vi "Check Large Range.vi"(8 "Tolerance":dbl=20.0, 9 "Differential Pressure":dbl, 10 "Diff Press Setpoint":dbl) -> (1 "In Range?":bool)   [LabVIEW 2018]
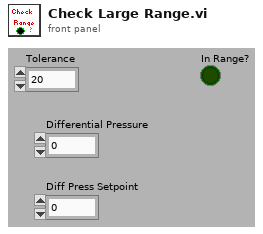
[diagram p1: front panel]
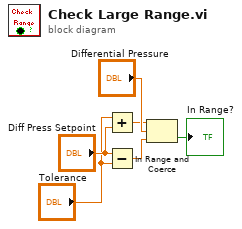
[diagram p0: block diagram]
diagram:
  n1 = Add(x="Tolerance", y="Diff Press Setpoint") -> (x+y=w2:dbl)
  n2 = Subtract(x="Diff Press Setpoint", y="Tolerance") -> (x-y=w3:dbl)
  n3 = In Range and Coerce(upper limit=w2, x="Differential Pressure", lower limit=w3) -> (In Range?=→"In Range?":bool)  [unwired: 1 out]
